vi "HitrapGUI.panel.vi"(0 "object ref":refnum<vi>, 5 "error in (no error)":errorcluster) -> (19 "error out":errorcluster)   [LabVIEW 2014, in "HitrapGUI.lvlib"]
doc: "This is the main GUI for the HITRAP facility\n\ndescriptionHelpStart\nThis is the main GUI for the HITRAP facility\ndescriptionHelpStop\n\naboutHelpStart\nLicense Agreement for this software:\n\nCopyright (C) 2009 Dietrich Beck\nGSI Helmholtzzentrum für Schwerionenforschung GmbH\nPlanckstraße 1\nD-64291 Darmstadt\nGermany\n\nContact: d.beck@gsi.de \n\nThis program is free software: you can redistribute it and/or modify it under the terms of the GNU General Public License as published by the Free Software Foundation, either version 3 of the License, or (at your option) any later version.\n\nThis program is distributed in the hope that it will be useful, but WITHOUT ANY WARRANTY; without even the implied warranty of MERCHANTABILITY or FITNESS FOR A PARTICULAR PURPOSE. See the GNU General Public License for more details.\n\nYou should have received a copy of the GNU General Public License along with this program.\nIf not, see <http://www.gnu.org/licenses/>.\n\nFor all questions and ideas contact: d.beck@gsi.de\nLast update: 18-MAR-2010\naboutHelpStop\n\nmenuHelpStart\nexplain menu here...\nmenuHelpStop"
uses:
  HitrapGUI.lvlib
  CSlibraries/GUILib/GUILib.userEventsMainType.ctl
  CSCore/BaseProcess/BaseProcess.descriptor string definition.ctl
  CSlibraries/UtilityLib/UtilityLib.valueStatus.ctl
  CSlibraries/UtilityLib/UtilityLib.helpType.ctl
  CSCore/CSSystem/CoreLib/CoreLib.string 2 byte array.vi
  CSCore/CSSystem/CoreLib/CoreLib.short 2 byte array.vi
  CSCore/CSSystem/CSSystemLib/CSSystemLib.lvlib
  CSlibraries/UtilityLib/UtilityLib.lvlib
  CSlibraries/GUILib/GUILib.lvlib
  CSCore/BaseProcess/BaseProcess.lvlib
  CSCore/CSSystem/CoreLib/CoreLib.lvlib
  CSCore/GUIs/GOGControllerGUI/GOGControllerGUI.lvlib
panel:
  in  "topSystem":bool
  in  "configID":string
  out "subSystem5StateQuality":string
  out "subSystem5State":string
  out "subSystem4StateQuality":string
  out "subSystem4State":string
  out "subSystem3StateQuality":string
  out "subSystem3State":string
  out "subSystem2StateQuality":string
  out "subSystem2State":string
  out "subSystem1StateQuality":string
  out "subSystem1State":string
  in  "Manuel Selection":T1(radio)
  out "Manual Control":string[][](table)=[["TR6ME1", "0", "0"], ["TR6KX1", "0", "0"], ["TR6KY1", "0", "0"], ["TR6QD1_1", "0", "0"], ["TR6QD1_2", "0", "0"], ["TR6MU1", "0", "0"], ["TR6QT1_1", "0", "0"], ["TR6QT1_2", "0", "0"], ["TR6QT1_3", "0", "0"], ["TR6KX2", "0", "0"], ["TR6KY2", "0", "0"], ["TR6KX3", "0", "0"], ["TR6KY3", "0", "0"], ["TR6QD2_1", "0", "0"], ["TR6QD2_2", "0", "0"], ["TR6QD3_1", "0", "0"], ["TR6QD3_2", "0", "0"]]
  in  "Oscilloscope Button":bool
  in  "Keithley Button":bool
  in  "IMAQ Button":bool
  out "versionInfo":string
  out "facilityName":string
  out "timeAndDate":string
  out "subSystem6State":string
  out "subSystem6StateQuality":string
  in  "focus":u16(ring) items=["COMPLETE", "Office9", "MM6", "FPGA-MCS", "HVSwitches", "AnalogHV", "Vorort6b", "Vorort6", "PB_DIO", "OPCGateway", "VorortCam", "Vorort4", "DAQMIO", "FPGA", "CANTest", "Vorort2", "TestSystem", "TestSystem71", "DSCBackend", "Labor2", "LxTest", "Office11", "RTTest"]
  out "focusColor":string
  out "mainSystemStateQuality":string
  out "actualSystemName":string
  out "mainSystemState":string
  in  "GOGFrontPanel.i attribute":T3
  out "# unack alarm":i32
  out "errorString":string
  out "errorFlag":bool
  out "infoStatus4":string
  out "errorGUI":string
  out "mainSystemName":string
  in  "next":bool
  in  "previous":bool
  in  "errorType":errorcluster
  in  "include":bool
  in  "exclude":bool
  out "infoStatus3":string
  in  "userEventsMain":T4
  in  "userEventsMainType":T4
  # "Top"
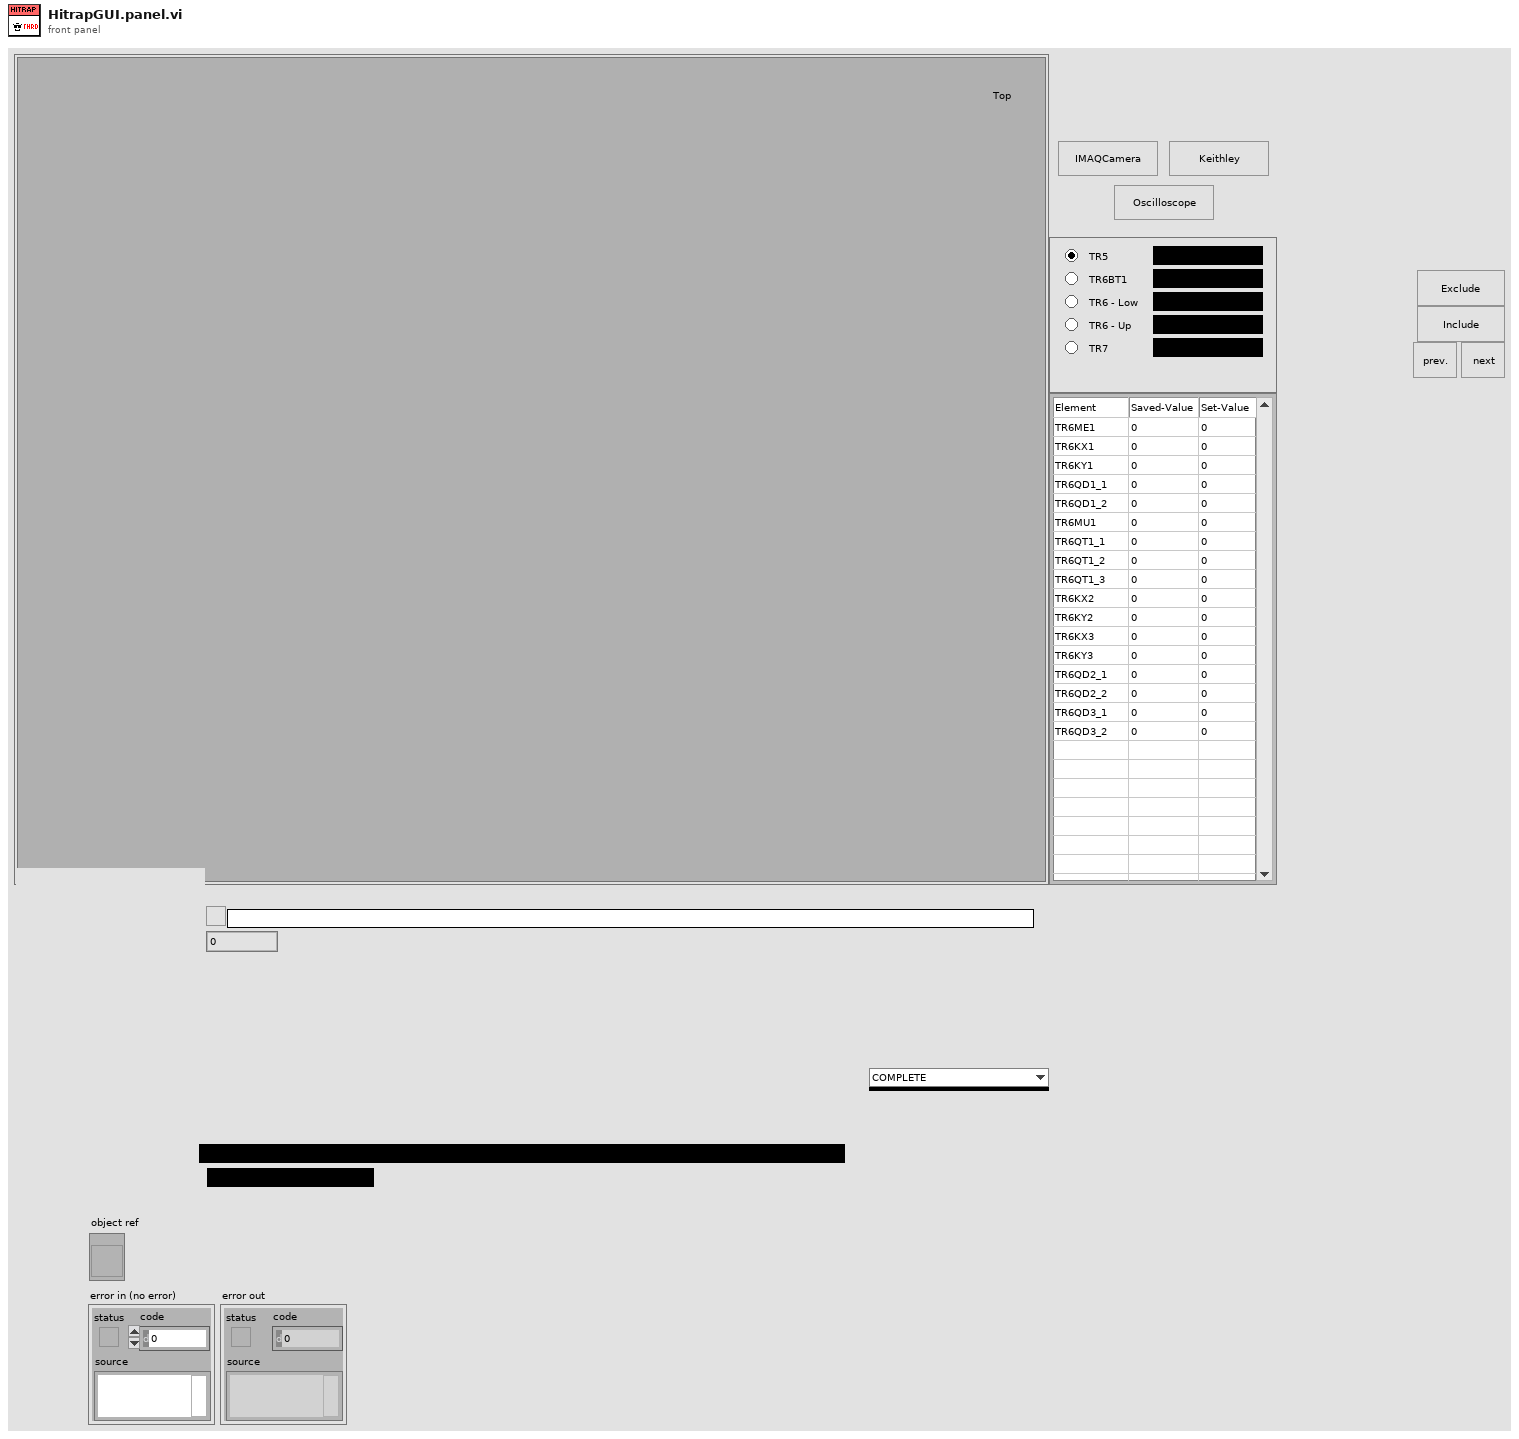
[diagram p1: front panel]
types:
  T1 = enum32{"Radio Selection 1", "Radio Selection 2", "Radio Selection 3", "Radio Selection 4", "Radio Selection 5"}
  T2 = typedef "BaseProcess.lvlib/BaseProcess.descriptor string definition.ctl" = string
  T3 = cluster{"GOGObject":string, "Object":string, "Method":string, "Descriptor":T2, "Input Descriptor":string, "Output Descriptor":string, "inputNames":string[], "outputNames":string[], "Values":cluster{"descriptor":string, "value":string}[]}
  T4 = typedef "GUILib.lvlib/GUILib.userEventsMainType.ctl" = cluster{"data":string, "dataType":i32}
  T5 = typedef "UtilityLib.lvlib/UtilityLib.valueStatus.ctl" = enum16{"no info available", "stand by/off", "on", "warning", "alarm/malfunction", "not implemented", "user action required", "important information", "system default", "control default", "indicator default", "button default"}
  T6 = typedef "UtilityLib.lvlib/UtilityLib.helpType.ctl" = enum16{"unknown", "menu", "description", "about", "special0", "special1", "special2"}
  T7 = typedef "CoreDefs.rawDataType.ctl" = i8[]
  T8 = typedef "HitrapGUI.lvlib/HitrapGUI.i attribute.ctl" = cluster{"SVs":refnum<k21>[], "DSCIntProc":string, "MotorActivityID":i32}
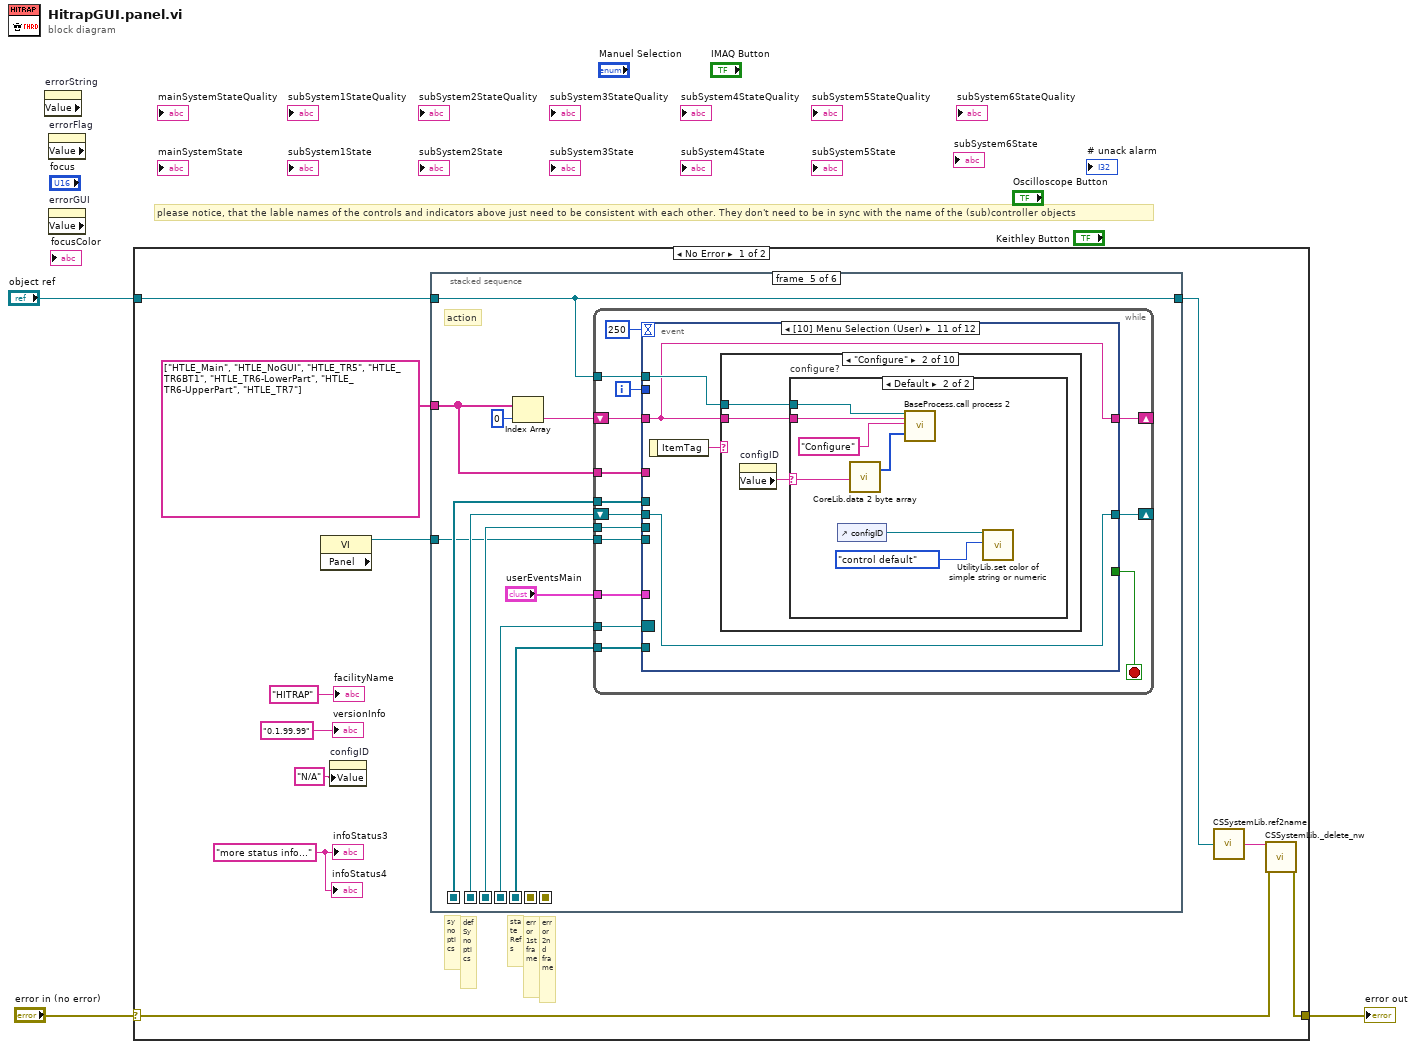
[diagram p0: block diagram]
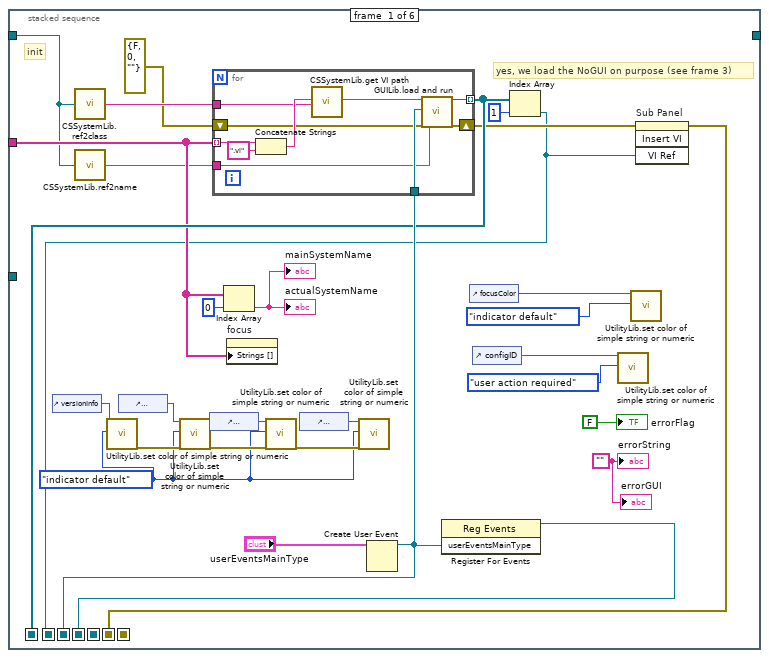
[diagram p2: hidden frame]
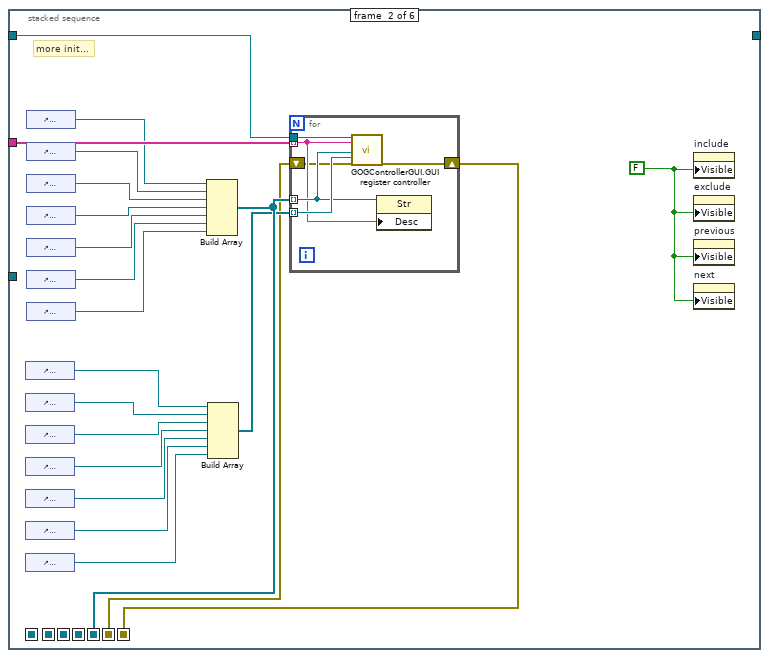
[diagram p3: hidden frame]
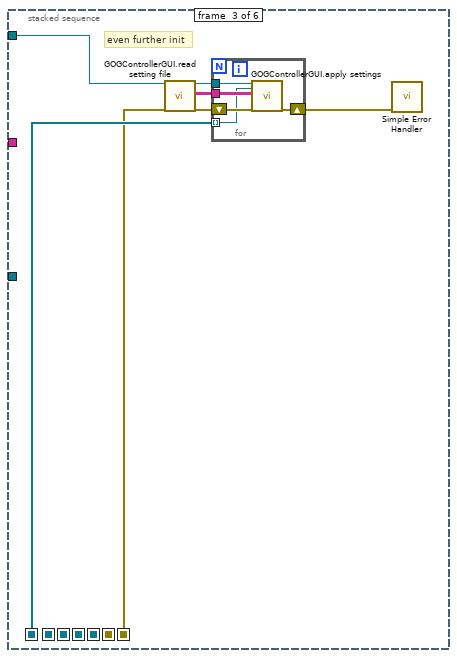
[diagram p4: hidden frame]
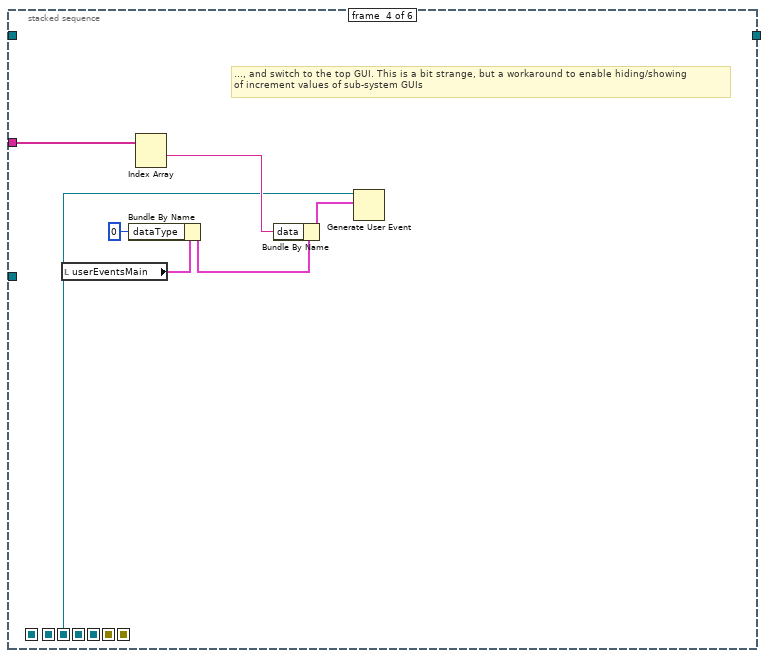
[diagram p5: hidden frame]
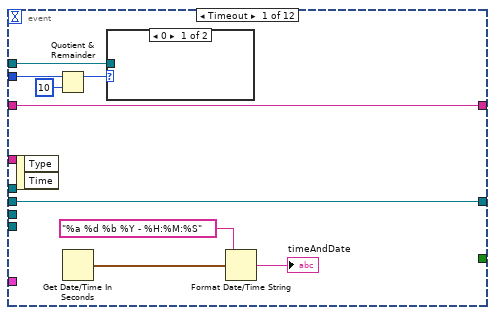
[diagram p6: hidden frame]
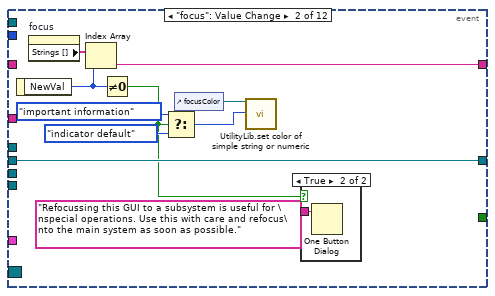
[diagram p8: hidden frame]
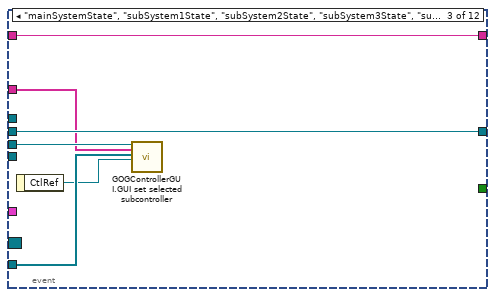
[diagram p10: hidden frame]
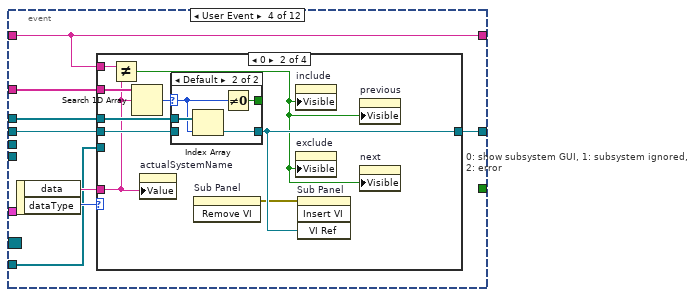
[diagram p11: hidden frame]
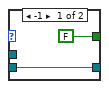
[diagram p13: hidden frame]
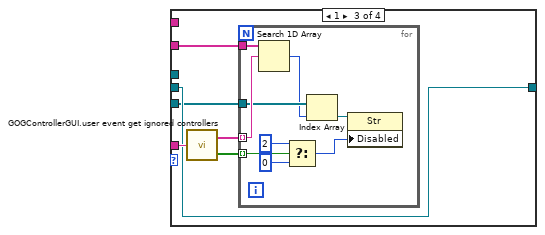
[diagram p14: hidden frame]
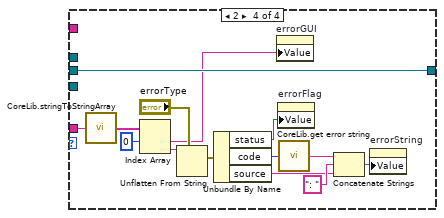
[diagram p15: hidden frame]
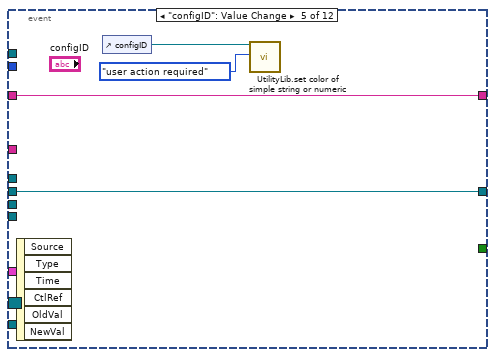
[diagram p16: hidden frame]
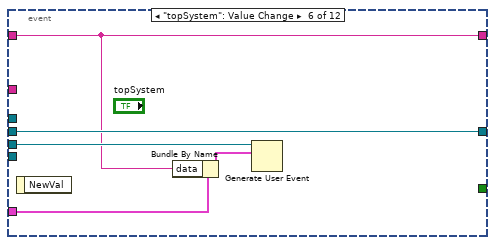
[diagram p17: hidden frame]
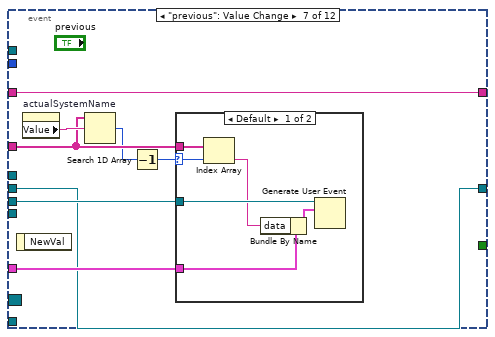
[diagram p18: hidden frame]
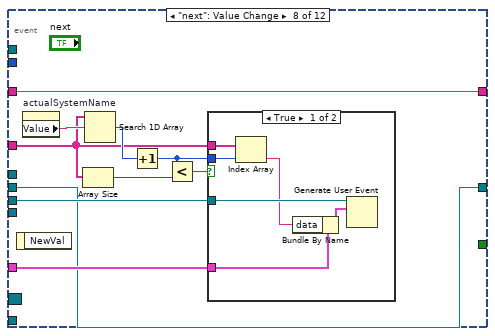
[diagram p20: hidden frame]
diagram:
  # "please notice, that the lable names of the controls and indicators above just need to be consistent with each other. They don't need to be in sync with the name of the (sub)controller objects"
  n1 = property on="errorString" class="Str" props=["Value"]() -> ()  [unwired: 2 in, 3 out]
  n2 = property on="errorFlag" class="Bool (strict)" props=["Value"]() -> ()  [unwired: 2 in, 3 out]
  n3 = property on="errorGUI" class="Str" props=["Value"]() -> ()  [unwired: 2 in, 3 out]
  n4 = case shown="No Error" "error in (no error)" {
    selector: "error in (no error)" -> [w12 w337]
    tunnel: [w14 w337] -> w2
    tunnel: "object ref" -> [w7 _]
    frame No Error {
      w11 = "more status info..." ("info1")
      # "error 2nd frame"
      # "error 1st frame"
      # "stateRefs"
      # "defSynoptics"
      # "synoptics"
      n5 = property class="VI" props=["Panel"]() -> (reference out=w5:refnum<vi>)  [unwired: 2 in, 2 out]
      n6 = property on="configID" class="Str"("Value"="N/A" ("configID")) -> ()  [unwired: 2 in, 2 out]
      n7 = stacked-sequence {
        seq-local: [w40 _ _ _ _ _] -> [_ _ w83 _ w108 w319]
        seq-local: [w43 _ _ _ _ _] -> [_ _ _ _ w110 w324]
        seq-local: [w41 _ _ _ _ _] -> [_ _ _ w95 w107 w322]
        seq-local: [w20 _ _ _ _ _] -> [_ _ _ _ w109 _]
        seq-local: [_ w71 _ _ _ _] -> [_ _ _ _ w101 _]
        seq-local: [w21 _ _ _ _ _] -> [_ w66 _ _ _ _]
        seq-local: [_ w65 _ _ _ _] -> [_ _ w82 _ _ _]
        tunnel: string[] ["HTLE_Main", "HTLE_NoGUI", "HTLE_TR5", "HTLE_TR6BT1", "HTLE_TR6-LowerPart", "HTLE_TR6-UpperPart", "HTLE_TR7"] -> [w30 w74 _ w97 w104 _]
        tunnel: w7 -> [w25 w67 w84 _ w105 _]
        tunnel: [_ _ _ _ w105 _] -> w6
        tunnel: w5 -> [_ _ _ _ w106 _]
        frame #0 {
          w26 = "" ("errorString")
          w17 = UtilityLib.valueStatus."indicator default" ("valueStatus")
          # "yes, we load the NoGUI on purpose (see frame 3)"
          # "init"
          n8 = control-ref of="versionInfo"() -> (w15:refnum<vi>)
          n9 = call "CSSystemLib.ref2class.vi"("obj refnum"=w25) -> ("class"=w33:string)
          n10 = call "CSSystemLib.ref2name.vi"("obj refnum"=w25) -> ("name"=w24:string)
          n11 = call "UtilityLib.set color of simple string or numeric.vi"("simpleString"=w15, "valueStatus"=w17) -> ("error out"=w18:errorcluster)  [unwired: 17 in]
          n12 = control-ref of="facilityName"() -> (w16:refnum<vi>)
          n13 = call "UtilityLib.set color of simple string or numeric.vi"("simpleString"=w16, "valueStatus"=w17, "error in (no error)"=w18) -> ("error out"=w19:errorcluster)  [unwired: 16 in]
          n14 = control-ref of="timeAndDate"() -> (w37:refnum<vi>)
          n15 = Index Array(array=w30, index=0) -> (element=→"actualSystemName" →"mainSystemName":string)
          n16 = property on="focus" class="Ring (strict)"("Strings []"=w30) -> ()  [unwired: 2 in, 2 out]
          n17 = call "UtilityLib.set color of simple string or numeric.vi"("simpleString"=w37, "valueStatus"=w17, "error in (no error)"=w19) -> ("error out"=w35:errorcluster)  [unwired: 16 in]
          n18 = control-ref of="actualSystemName"() -> (w36:refnum<vi>)
          n19 = call "UtilityLib.set color of simple string or numeric.vi"("simpleString"=w36, "valueStatus"=w17, "error in (no error)"=w35) -> ()  [unwired: 16 in, 1 out]
          n20 = Create User Event(user event datatype="userEventsMainType") -> (user event=w41:refnum<user-event>)  [unwired: 1 in, 1 out]
          n21 = for {
            tunnel: [w53] -> w40 mode=indexing
            tunnel: w41 -> [w49]
            tunnel: w30 -> [w52] mode=indexing
            tunnel: w33 -> [w47]
            tunnel: w24 -> [w48]
            shift-right: [w45] -> w22
            shift-left: errorcluster {"status"=FALSE, "code"=0, "source"=""} ("error in (no error)") -> [w46]
            n22 = Concatenate Strings(w52, ".vi" ("string")) -> (w50:string)
            n23 = call "CSSystemLib.get VI path.vi"("method"=w50, "class"=w47) -> ("VI path"=w44:string)  [unwired: 15 in, 2 out]
            n24 = call "GUILib.load and run.vi"("path"=w44, "userEvent"=w49, "error in (no error)"=w46, "iniData"=w48) -> ("VIRef"=w53:refnum<vi>, "error out"=w45:errorcluster)  [unwired: 14 in]
          }
          n25 = register-events(w41) -> (reference out=w43:refnum<event-registration>)  [unwired: 2 in, 1 out]
          n26 = control-ref of="focusColor"() -> (w29:refnum<vi>)
          n27 = control-ref of="configID"() -> (w32:refnum<vi>)
          n28 = Index Array(array=w40, index=1) -> (element=w20:refnum<vi>)
          n29 = call "UtilityLib.set color of simple string or numeric.vi"("simpleString"=w32, "valueStatus"=UtilityLib.valueStatus."user action required") -> ()  [unwired: 17 in, 1 out]
          n30 = call "UtilityLib.set color of simple string or numeric.vi"("simpleString"=w29, "valueStatus"=UtilityLib.valueStatus."indicator default") -> ()  [unwired: 17 in, 1 out]
          n31 = invoke on="Sub Panel" class="SubPnl" method="Insert VI"(error in=w22, "VI Ref"=w20) -> (error out=w21:errorcluster)  [unwired: 2 in, 3 out]
          "errorFlag" <- FALSE ("errorFlag")
          "errorString" <- w26
          "errorGUI" <- w26
        }
        frame #1 {
          w56 = FALSE ("Visible")
          # "more init..."
          n32 = control-ref of="mainSystemStateQuality"() -> (w69:refnum<vi>)
          n33 = control-ref of="subSystem1StateQuality"() -> (w70:refnum<vi>)
          n34 = control-ref of="subSystem2StateQuality"() -> (w62:refnum<vi>)
          n35 = control-ref of="subSystem3StateQuality"() -> (w61:refnum<vi>)
          n36 = control-ref of="subSystem4StateQuality"() -> (w58:refnum<vi>)
          n37 = control-ref of="subSystem5StateQuality"() -> (w57:refnum<vi>)
          n38 = control-ref of="subSystem6StateQuality"() -> (w54:refnum<vi>)
          n39 = control-ref of="mainSystemState"() -> (w73:refnum<vi>)
          n40 = control-ref of="subSystem1State"() -> (w72:refnum<vi>)
          n41 = control-ref of="subSystem2State"() -> (w64:refnum<vi>)
          n42 = control-ref of="subSystem3State"() -> (w63:refnum<vi>)
          n43 = control-ref of="subSystem4State"() -> (w60:refnum<vi>)
          n44 = control-ref of="subSystem5State"() -> (w59:refnum<vi>)
          n45 = control-ref of="subSystem6State"() -> (w55:refnum<vi>)
          n46 = Build Array(w73, w72, w64, w63, w60, w59, w55) -> (w71:refnum<vi>[])
          n47 = Build Array(w69, w70, w62, w61, w58, w57, w54) -> (w68:refnum<vi>[])
          n48 = for {
            tunnel: w71 -> [w78] mode=indexing
            tunnel: w74 -> [w77] mode=indexing
            tunnel: w68 -> [w79] mode=indexing
            tunnel: w67 -> [w80]
            shift-right: [w75] -> w65
            shift-left: w66 -> [w76]
            n49 = call "GOGControllerGUI.GUI register controller.vi"("i ref in"=w80, "controllerName"=w77, "subSystemState"=w78, "subSystemStateQuality"=w79, "error in (no error)"=w76) -> ("error out"=w75:errorcluster)  [unwired: 13 in, 1 out]
            n50 = property class="Str"(reference=w78, "Desc"=w77) -> ()  [unwired: 1 in, 2 out]
          }
          n51 = property on="include" class="Bool"("Visible"=w56) -> ()  [unwired: 2 in, 2 out]
          n52 = property on="exclude" class="Bool"("Visible"=w56) -> ()  [unwired: 2 in, 2 out]
          n53 = property on="previous" class="Bool"("Visible"=w56) -> ()  [unwired: 2 in, 2 out]
          n54 = property on="next" class="Bool"("Visible"=w56) -> ()  [unwired: 2 in, 2 out]
        }
        frame #2 {
          # "even further init"
          n55 = call "GOGControllerGUI.read setting file.vi"("i ref in"=w84, "error in (no error)"=w82) -> ("i ref out"=w87:refnum<vi>, "deviceArray"=w86:string[][], "error out"=w85:errorcluster)  [unwired: 15 in]
          n56 = for {
            tunnel: w87 -> [w92]
            tunnel: w86 -> [w91]
            tunnel: w83 -> [w89] mode=indexing
            shift-right: [w88] -> w81
            shift-left: w85 -> [w90]
            n57 = call "GOGControllerGUI.apply settings.vi"("i ref in"=w92, "GUIRef"=w89, "deviceArray"=w91, "error in (no error)"=w90) -> ("error out"=w88:errorcluster)  [unwired: 14 in, 1 out]
          }
          n58 = call <vilib>:"Simple Error Handler.vi"("error in (no error)"=w81) -> ()  [unwired: 4 in, 5 out]
        }
        frame #3 {
          # "..., and switch to the top GUI. This is a bit strange, but a workaround to enable hiding/showing\nof increment values of sub-system GUIs"
          n59 = local read "userEventsMain"() -> (w99:T4)
          n60 = Bundle By Name(cluster=w99, "dataType"=0) -> (w94:T4)
          n61 = Index Array(array=w97) -> (element #1=w96:string)  [unwired: 2 in, 1 out]
          n62 = Bundle By Name(cluster=w94, "data"=w96) -> (w93:T4)
          n63 = Generate User Event(user event=w95, event data cluster=w93) -> ()  [unwired: 2 in, 2 out]
        }
        frame #4 {
          # "action"
          n64 = Index Array(array=w104, index=0) -> (element=w102:string)
          n65 = while {
            tunnel: w110 -> [w124]
            shift-right: [w123] -> _
            shift-left: w109 -> [w122]
            tunnel: w104 -> [w121]
            tunnel: w108 -> [w120]
            tunnel: w107 -> [w119]
            tunnel: w106 -> [w117]
            tunnel: w105 -> [w116]
            shift-right: [w114] -> _
            shift-left: w102 -> [w115]
            tunnel: w101 -> [w113]
            tunnel: "userEventsMain" -> [w112]
            i -> [w111]
            stop <- w125 stop-if-true
            n66 = event shown="[10] Menu Selection (User)" {
              selector: w124 -> [_ _ _ _ _ _ _ _ _ _ _ _]
              dyn-events: _ -> [_ _ _ _ _ _ _ _ _ _ _ _]
              timeout: 250 -> [_ _ _ _ _ _ _ _ _ _ _ _]
              tunnel: [_ _ _ _ _ _ _ _ _ _ _ w316] -> w125
              tunnel: [w134 w142 w151 w157 w208 w213 w215 w232 w248 w275 w280 w315] -> w123
              tunnel: w122 -> [w134 w142 w151 w159 w208 w213 w215 w232 w248 w275 w280 w315]
              tunnel: w121 -> [_ _ w146 w155 _ _ w217 w231 w260 _ _ _]
              tunnel: w120 -> [_ _ _ w158 _ _ _ _ w246 _ _ _]
              tunnel: w119 -> [_ _ w149 _ _ w212 w221 w237 _ _ _ _]
              tunnel: w117 -> [_ _ _ _ _ _ _ _ _ _ _ _]
              tunnel: w116 -> [w126 _ _ _ _ _ _ _ w261 w268 w278 _]
              tunnel: w115 -> [w130 _ w150 w152 w205 w210 w220 w236 w253 w276 w277 w314]
              tunnel: [w130 w144 w150 w152 w205 w210 w220 w236 w253 w276 w277 w314] -> w114
              tunnel: w113 -> [_ _ w148 w153 _ _ _ _ _ _ _ _]
              tunnel: w112 -> [_ _ _ _ _ w209 w219 w235 _ _ _ _]
              tunnel: w111 -> [w129 _ _ _ _ _ _ _ _ _ _ _]
              event Timeout {
                n67 = event-data() -> ()  [unwired: 1 in, 2 out]
                n68 = Quotient & Remainder(x=w129, y=10) -> (x-y*floor(x/y)=w127:i32)  [unwired: 1 out]
                n69 = Get Date/Time In Seconds() -> (seconds since 1Jan1904=w133:timestamp)
                n70 = case shown="0" w127 {
                  tunnel: w126 -> [_ _]
                  frame 0 {
                  }
                  frame Default {
                  }
                }
                n71 = Format Date/Time String(time format string (%c)="%a %d %b %Y - %H:%M:%S", seconds (now)=w133) -> (date/time string=→"timeAndDate":string)  [unwired: 1 in]
              }
              event "focus": Value Change {
                n72 = event-data() -> ("NewVal"=w141:u16)  [unwired: 1 in]
                n73 = property on="focus" class="Ring (strict)"() -> ("Strings []"=w143:string[])  [unwired: 2 in, 2 out]
                n74 = Index Array(array=w143, index=w141) -> (element=w144:string)
                n75 = Not Equal To 0?(x=w141) -> (x != 0?=w135:bool)
                n76 = Select(t=UtilityLib.valueStatus."important information", s=w135, f=UtilityLib.valueStatus."indicator default" ("State")) -> (s? t:f=w137:T5)
                n77 = control-ref of="focusColor"() -> (w138:refnum<vi>)
                n78 = call "UtilityLib.set color of simple string or numeric.vi"("simpleString"=w138, "valueStatus"=w137) -> ()  [unwired: 17 in, 1 out]
                n79 = case shown="True" w135 {
                  tunnel: "Refocussing this GUI to a subsystem is useful for \nspecial operations. Use this with care and refocus\nto the main system as soon as possible." ("message") -> [_ w145]
                  frame False {
                  }
                  frame True {
                    n80 = One Button Dialog(message=w145) -> ()  [unwired: 1 in, 1 out]
                  }
                }
              }
              event "mainSystemState", "subSystem1State", "subSystem2State", "subSystem3State", "subSystem4State", "subSystem5State", "subSystem6State": Mouse Down {
                n81 = event-data() -> ("CtlRef"=w147:refnum<vi>)  [unwired: 1 in]
                n82 = call "GOGControllerGUI.GUI set selected subcontroller.vi"("userEvent"=w149, "controllerNames"=w146, "controllerRefs"=w148, "controllerRef"=w147) -> ()  [unwired: 16 in]
              }
              event User Event {
                n83 = event-data() -> ("data"=w156:string, "dataType"=w154:i32)  [unwired: 1 in]
                n84 = case "0: show subsystem GUI, 1: subsystem ignored, 2: error" shown="0" w154 {
                  tunnel: w159 -> [w160 w169 w180 w204]
                  tunnel: w158 -> [_ w167 _ _]
                  tunnel: [w160 w163 w180 w204] -> w157
                  tunnel: w156 -> [_ w164 w181 w203]
                  tunnel: w155 -> [_ w166 w179 _]
                  tunnel: w153 -> [_ _ w176 _]
                  tunnel: w152 -> [_ w165 _ _]
                  frame Default {
                  }
                  frame 0 {
                    n85 = Not Equal?(x=w165, y=w164) -> (x != y?=w161:bool)
                    n86 = Search 1D Array(1D array=w166, element=w164) -> (index of element=w168:i32)  [unwired: 1 in]
                    n87 = property on="actualSystemName" class="Str"("Value"=w164) -> ()  [unwired: 2 in, 2 out]
                    n88 = case shown="Default" w168 {
                      selector: w168 -> [_ w173]
                      tunnel: [w171 w174] -> w163
                      tunnel: w169 -> [w171 _]
                      tunnel: w167 -> [_ w175]
                      tunnel: [FALSE w172] -> _
                      frame -1 {
                      }
                      frame Default {
                        n89 = Index Array(array=w175, index=w173) -> (element=w174:refnum<vi>)
                        n90 = Not Equal To 0?(x=w173) -> (x != 0?=w172:bool)
                      }
                    }
                    n91 = invoke on="Sub Panel" class="SubPnl" method="Remove VI"() -> (error out=w162:errorcluster)  [unwired: 3 in, 2 out]
                    n92 = property on="include" class="Bool"("Visible"=w161) -> ()  [unwired: 2 in, 2 out]
                    n93 = property on="exclude" class="Bool"("Visible"=w161) -> ()  [unwired: 2 in, 2 out]
                    n94 = invoke on="Sub Panel" class="SubPnl" method="Insert VI"(error in=w162, "VI Ref"=w163) -> ()  [unwired: 2 in, 4 out]
                    n95 = property on="previous" class="Bool"("Visible"=w161) -> ()  [unwired: 2 in, 2 out]
                    n96 = property on="next" class="Bool"("Visible"=w161) -> ()  [unwired: 2 in, 2 out]
                  }
                  frame 1 {
                    n97 = call "GOGControllerGUI.user event get ignored controllers.vi"("data"=w181) -> ("controllers"=w178:string[], "ignored"=w177:bool[])
                    n98 = for {
                      tunnel: w179 -> [w190]
                      tunnel: w178 -> [w189] mode=indexing
                      tunnel: w177 -> [w188] mode=indexing
                      tunnel: w176 -> [w185]
                      n99 = Search 1D Array(1D array=w190, element=w189) -> (index of element=w184:i32)  [unwired: 1 in]
                      n100 = Select(t=2, s=w188, f=0) -> (s? t:f=w182:i32)
                      n101 = Index Array(array=w185, index=w184) -> (element=w183:refnum<vi>)
                      n102 = property class="Str"(reference=w183, "Disabled"=w182) -> ()  [unwired: 1 in, 2 out]
                    }
                  }
                  frame 2 {
                    n103 = call "CoreLib.stringToStringArray.vi"("String"=w203) -> ("Array"=w202:string[])
                    n104 = Index Array(array=w202, index #1=0 ("index")) -> (element #1=w191:string, element #2=w200:string)  [unwired: 1 in]
                    n105 = Unflatten From String(type="errorType", binary string=w200) -> (value=w198:errorcluster)  [unwired: 3 in, 2 out]
                    n106 = Unbundle By Name(w198) -> ("status"=w196:bool, "code"=w197:i32, "source"=w193:string)
                    n107 = property on="errorGUI" class="Str"("Value"=w191) -> ()  [unwired: 2 in, 2 out]
                    n108 = property on="errorFlag" class="Bool (strict)"("Value"=w196) -> ()  [unwired: 2 in, 2 out]
                    n109 = call "CoreLib.get error string.vi"("Error Code"=w197) -> ("Error String"=w195:string)
                    n110 = Concatenate Strings(w195, ": " ("string"), w193) -> (w192:string)
                    n111 = property on="errorString" class="Str"("Value"=w192) -> ()  [unwired: 2 in, 2 out]
                  }
                }
              }
              event "configID": Value Change {
                n112 = event-data() -> ()  [unwired: 1 in, 6 out]
                n113 = control-ref of="configID"() -> (w207:refnum<vi>)
                n114 = call "UtilityLib.set color of simple string or numeric.vi"("simpleString"=w207, "valueStatus"=UtilityLib.valueStatus."user action required") -> ()  [unwired: 17 in, 1 out]
              }
              event "topSystem": Value Change {
                n115 = event-data() -> ()  [unwired: 1 in, 1 out]
                n116 = Bundle By Name(cluster=w209, "data"=w210) -> (w211:T4)
                n117 = Generate User Event(user event=w212, event data cluster=w211) -> ()  [unwired: 2 in, 2 out]
              }
              event "previous": Value Change {
                n118 = event-data() -> ()  [unwired: 1 in, 1 out]
                n119 = property on="actualSystemName" class="Str"() -> ("Value"=w218:string)  [unwired: 2 in, 2 out]
                n120 = Search 1D Array(1D array=w217, element=w218) -> (index of element=w216:i32)  [unwired: 1 in]
                n121 = Decrement(x=w216) -> (x-1=w214:i32)
                n122 = case shown="Default" w214 {
                  selector: w214 -> [w222 _]
                  tunnel: w221 -> [w227 _]
                  tunnel: w219 -> [w225 _]
                  tunnel: w217 -> [w224 _]
                  frame Default {
                    n123 = Index Array(array=w224, index=w222) -> (element=w223:string)
                    n124 = Bundle By Name(cluster=w225, "data"=w223) -> (w226:T4)
                    n125 = Generate User Event(user event=w227, event data cluster=w226) -> ()  [unwired: 2 in, 2 out]
                  }
                  frame -1, 0 {
                  }
                }
              }
              event "next": Value Change {
                n126 = event-data() -> ()  [unwired: 1 in, 1 out]
                n127 = property on="actualSystemName" class="Str"() -> ("Value"=w234:string)  [unwired: 2 in, 2 out]
                n128 = Array Size(array=w231) -> (size(s)=w230:i32)
                n129 = Search 1D Array(1D array=w231, element=w234) -> (index of element=w233:i32)  [unwired: 1 in]
                n130 = Increment(x=w233) -> (x+1=w228:i32)
                n131 = Less?(x=w228, y=w230) -> (x < y?=w229:bool)
                n132 = case shown="True" w229 {
                  tunnel: w237 -> [w243 _]
                  tunnel: w235 -> [w241 _]
                  tunnel: w231 -> [w240 _]
                  tunnel: w228 -> [w238 _]
                  frame True {
                    n133 = Index Array(array=w240, index=w238) -> (element=w239:string)
                    n134 = Bundle By Name(cluster=w241, "data"=w239) -> (w242:T4)
                    n135 = Generate User Event(user event=w243, event data cluster=w242) -> ()  [unwired: 2 in, 2 out]
                  }
                  frame False {
                  }
                }
              }
              event "exclude", "include": Value Change {
                w244 = 0
                n136 = event-data() -> ("CtlRef"=w252:refnum<vi>)  [unwired: 1 in]
                n137 = control-ref of="exclude"() -> (w250:refnum<vi>)
                n138 = for {
                  tunnel: w246 -> [w265] mode=indexing
                  tunnel: [w264] -> w245 mode=indexing
                  tunnel: w244 -> [w263]
                  n139 = Type Cast(type=w263, x=w265) -> (*(type *) &x=w264:i32)
                }
                n140 = Type Cast(type=w244, x=w248) -> (*(type *) &x=w247:i32)
                n141 = Type Cast(type=w244, x=w252) -> (*(type *) &x=w251:i32)
                n142 = Type Cast(type=w244, x=w250) -> (*(type *) &x=w249:i32)
                n143 = Search 1D Array(1D array=w245, element=w247) -> (index of element=w262:i32)  [unwired: 1 in]
                n144 = Index Array(array=w260, index=w262) -> (element=w258:string)
                n145 = Equal?(x=w251, y=w249) -> (x = y?=w255:bool)
                n146 = call-poly "CoreLib.data 2 byte array.vi"("string"=w258) -> ("byteArray out"=w257:T7)  [unwired: 18 in]
                n147 = Boolean To (0,1)(Boolean=w255) -> (0, 1=w254:i16)
                n148 = call-poly "CoreLib.data 2 byte array.vi"("byteArray"=w257, "i16"=w254) -> ("byteArray out"=w256:T7)  [unwired: 17 in]
                n149 = call "BaseProcess.call process 2.vi"("i ref in"=w261, "Object"=w253, "Selector"="IgnoreSubController", "Data"=w256) -> ()  [unwired: 14 in, 2 out]
              }
              event "# unack alarm": Mouse Down {
                w270 = TRUE  # prefixSystemName
                n150 = event-data() -> ()  [unwired: 1 in, 7 out]
                n151 = call "HitrapGUI.get i attribute.vi"("i ref in"=w268) -> ("i attribute"=w267:T8)  [unwired: 16 in, 2 out]
                n152 = Unbundle By Name(w267) -> ("DSCIntProc"=w266:string)
                n153 = Bundle By Name(cluster="GOGFrontPanel.i attribute", "Object"=w266) -> (w273:T3)
                n154 = Flatten To String(anything=w273) -> (data string=w274:string)  [unwired: 3 in, 2 out]
                n155 = call "CSSystemLib._new_nw.vi"("objectName"="AlarmViewer" ("Data"), "prefixSystemName"=w270, "className"="DSCAlarmGUI", "data in"=w274) -> ()  [unwired: 13 in, 3 out]
              }
              event Menu Selection (User) {
                n156 = event-data() -> ("ItemTag"=w279:string)  [unwired: 1 in]
                n157 = case shown="\"Configure\"" w279 {
                  tunnel: w278 -> [_ w282 w291 w299 w302 w306 w308 _ _ _]
                  tunnel: w277 -> [_ w281 w292 w300 w303 w305 w309 _ _ _]
                  frame Default {
                  }
                  frame "Configure" {
                    n158 = property on="configID" class="Str"() -> ("Value"=w283:string)  [unwired: 2 in, 2 out]
                    n159 = case "configure?" shown="Default" w283 {
                      selector: w283 -> [_ w286]
                      tunnel: w282 -> [_ w290]
                      tunnel: w281 -> [_ w289]
                      frame "", "N/A" {
                      }
                      frame Default {
                        n160 = control-ref of="configID"() -> (w284:refnum<vi>)
                        n161 = call-poly "CoreLib.data 2 byte array.vi"("string"=w286) -> ("byteArray out"=w287:T7)  [unwired: 18 in]
                        n162 = call "BaseProcess.call process 2.vi"("i ref in"=w290, "Object"=w289, "Selector"="Configure", "Data"=w287) -> ()  [unwired: 14 in, 2 out]
                        n163 = call "UtilityLib.set color of simple string or numeric.vi"("simpleString"=w284, "valueStatus"=UtilityLib.valueStatus."control default") -> ()  [unwired: 17 in, 1 out]
                      }
                    }
                  }
                  frame "SaveConfig" {
                    n164 = property on="configID" class="Str"() -> ("Value"=w293:string)  [unwired: 2 in, 2 out]
                    n165 = case "configure?" shown="Default" w293 {
                      selector: w293 -> [_ w294]
                      tunnel: w291 -> [_ w298]
                      tunnel: w292 -> [_ w297]
                      frame "", "N/A" {
                      }
                      frame Default {
                        n166 = call-poly "CoreLib.data 2 byte array.vi"("string"=w294) -> ("byteArray out"=w295:T7)  [unwired: 18 in]
                        n167 = call "BaseProcess.call process 2.vi"("i ref in"=w298, "Object"=w297, "Selector"="SaveConfiguration", "Data"=w295) -> ()  [unwired: 14 in, 2 out]
                      }
                    }
                  }
                  frame "PFO" {
                    n168 = call "BaseProcess.call process 2.vi"("i ref in"=w299, "Object"=w300, "Selector"="PrepareForOperation") -> ()  [unwired: 15 in, 2 out]
                  }
                  frame "ANV" {
                    n169 = call "BaseProcess.call process 2.vi"("i ref in"=w302, "Object"=w303, "Selector"="ApplyNominalValues") -> ()  [unwired: 15 in, 2 out]
                  }
                  frame "Reset" {
                    n170 = call "BaseProcess.call process 2.vi"("i ref in"=w306, "Object"=w305, "Selector"="ResetStateMachine") -> ()  [unwired: 15 in, 2 out]
                  }
                  frame "Recover" {
                    n171 = call "BaseProcess.call process 2.vi"("i ref in"=w308, "Object"=w309, "Selector"="Recover") -> ()  [unwired: 15 in, 2 out]
                  }
                  frame "about" {
                    n172 = call "UtilityLib.show help.vi"("helpType"=UtilityLib.helpType."about") -> ()
                  }
                  frame "description" {
                    n173 = call "UtilityLib.show help.vi"("helpType"=UtilityLib.helpType."description") -> ()
                  }
                  frame "menu" {
                    n174 = call "UtilityLib.show help.vi"("helpType"=UtilityLib.helpType."menu") -> ()
                  }
                }
              }
              event Panel Close? {
                n175 = event-data() -> ()  [unwired: 1 in, 4 out]
                n176 = Two Button Dialog(message="Close GUI...") -> (T button?=w316:bool)  [unwired: 2 in]
                n177 = event-data("Discard?"=TRUE) -> ()  [unwired: 1 in, 1 out]
              }
            }
          }
        }
        frame #5 {
          # "deinit"
          n178 = flat-sequence {
            tunnel: [w326] -> w321
            tunnel: w319 -> [w325]
            tunnel: w321 -> [w333]
            tunnel: [w333] -> w320
            tunnel: w320 -> [w335]
            frame #0 {
              n179 = for {
                tunnel: [w331] -> w326 mode=indexing
                tunnel: w325 -> [w331] mode=indexing
                n180 = control-ref of="topSystem"() -> (w328:refnum<vi>)
                n181 = call "GUILib.find control by name.vi"("control name"="stop", "VIRef"=w331) -> ("controlRef"=w330:refnum<vi>)  [unwired: 16 in, 1 out]
                n182 = Type Cast(type=w328, x=w330) -> (*(type *) &x=w329:refnum<vi>)
                n183 = property class="Bool"(reference=w329, "Val(Sgnl)"=TRUE) -> ()  [unwired: 1 in, 2 out]
              }
            }
            frame #1 {
              n184 = Wait (ms)(milliseconds to wait=u32 2000) -> ()  [unwired: 1 out]
            }
            frame #2 {
              n185 = for {
                tunnel: w335 -> [w336] mode=indexing
                n186 = Close Reference(reference=w336) -> ()  [unwired: 1 in, 1 out]
              }
            }
          }
          n187 = Unregister For Events(event registration refnum=w324) -> (error out=w323:errorcluster)  [unwired: 1 in]
          n188 = Destroy User Event(user event=w322, error in=w323) -> ()  [unwired: 1 out]
        }
      }
      n189 = call "CSSystemLib.ref2name.vi"("obj refnum"=w6) -> ("name"=w13:string)
      n190 = call "CSSystemLib._delete_nw.vi"("objectName"=w13, "error in (no error)"=w12) -> ("error out"=w14:errorcluster)  [unwired: 17 in]
      "facilityName" <- "HITRAP" ("facilityName")
      "versionInfo" <- "0.1.99.99" ("actualSystemName 3")
      "infoStatus3" <- w11
      "infoStatus4" <- w11
    }
    frame Error {
    }
  }
  "error out" <- w2
